vi "Set Artificial Scrollbar.vi"(8 "error in (no error)":errorcluster, 9 "# Displayed Items":i32, 10 "Array Size":i32, 11 "Scrollbar in":refnum<vi>) -> (0 "error IO":errorcluster)   [LabVIEW 2021]
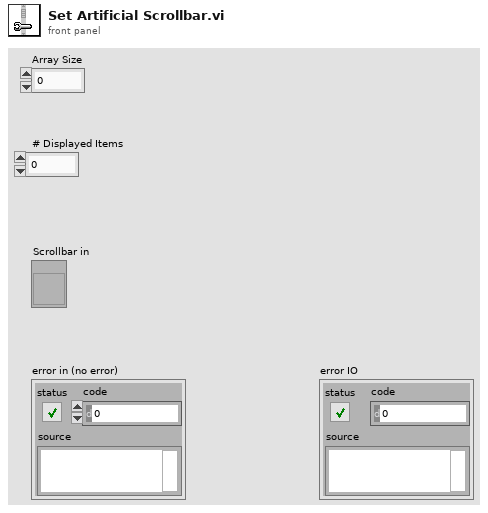
[diagram p1: front panel]
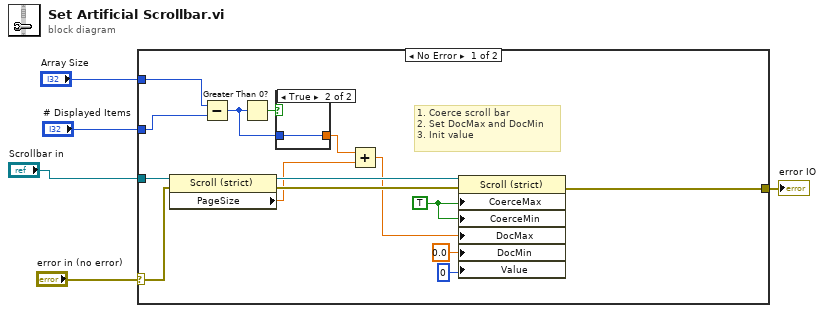
[diagram p0: block diagram]
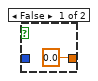
[diagram p2: hidden frame]
diagram:
  n1 = case shown="No Error" "error in (no error)" {
    selector: "error in (no error)" -> [w18 w23]
    tunnel: "Scrollbar in" -> [w20 _]
    tunnel: "Array Size" -> [w16 _]
    tunnel: "# Displayed Items" -> [w15 _]
    tunnel: [w9 w23] -> w2
    frame No Error {
      w13 = TRUE
      # "1. Coerce scroll bar\n2. Set DocMax and DocMin\n3. Init value"
      n2 = property class="Scroll (strict)"(reference=w20, error in=w18) -> (reference out=w19:refnum<vi>, error out=w17:errorcluster, "PageSize"=w14:dbl)
      n3 = Subtract(x=w16, y=w15) -> (x-y=w7:i32)
      n4 = Greater Than 0?(x=w7) -> (x > 0?=w8:bool)
      n5 = case shown="True" w8 {
        tunnel: w7 -> [_ w22]
        tunnel: [0.0 w22] -> w6
        frame False {
        }
        frame True {
        }
      }
      n6 = Add(x=w6, y=w14) -> (x+y=w11:dbl)
      n7 = property on="Property Node" class="Scroll (strict)"(reference=w19, error in=w17, "CoerceMax"=w13, "CoerceMin"=w13, "DocMax"=w11, "DocMin"=0.0 ("Doc Min"), "Value"=0) -> (error out=w9:errorcluster)  [unwired: 1 out]
    }
    frame Error {
    }
  }
  "error IO" <- w2
